vi "VNA_Save.vi"(2 "error in (no error)":errorcluster, 4 "File Path":string="C:\\NA_Measurements\\Temp\\test.s2p", 5 "VISA resource name":refnum<visa-resource-name>) -> (0 "error out":errorcluster, 1 "VISA resource out":refnum<visa-resource-name>)   [LabVIEW 2017]
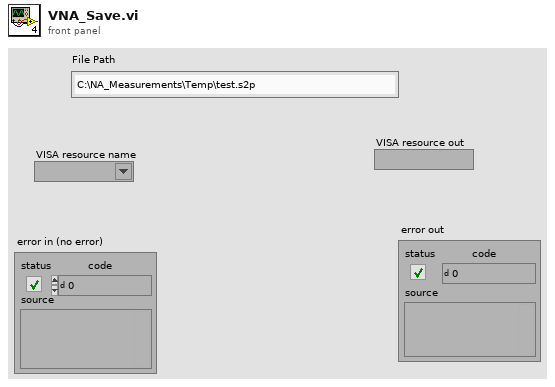
[diagram p1: front panel]
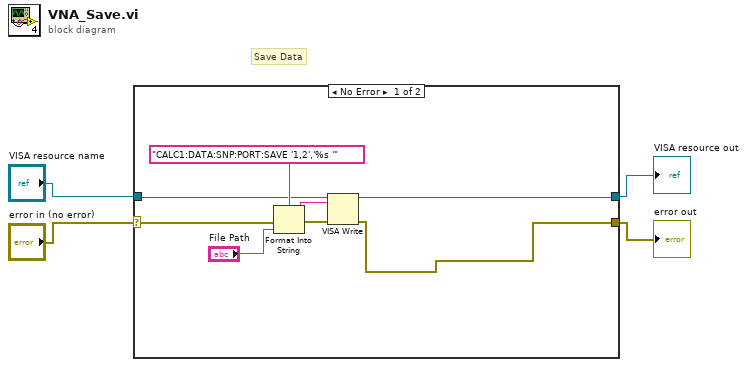
[diagram p0: block diagram]
diagram:
  # "Save Data"
  n1 = case shown="No Error" "error in (no error)" {
    selector: "error in (no error)" -> [w8 w14]
    tunnel: [w5 w14] -> w3
    tunnel: "VISA resource name" -> [w7 w13]
    tunnel: [w6 w13] -> w4
    frame No Error {
      n2 = Format Into String(format string="CALC1:DATA:SNP:PORT:SAVE '1,2','%s '" ("Cmdline"), error in=w8, "File Path") -> (resulting string=w12:string, error out=w11:errorcluster)  [unwired: 1 in]
      n3 = VISA Write(VISA resource name=w7, write buffer=w12, error in (no error)=w11) -> (VISA resource name out=w6:refnum<visa-resource-name>, error out=w5:errorcluster)  [unwired: 1 out]
    }
    frame Error {
    }
  }
  "error out" <- w3
  "VISA resource out" <- w4
